vi "ToDatagram.vi"(8 "error in (no error)":errorcluster, 10 "messageID":u16, 11 "BaseMqttMsg in":refnum<class "BaseMqttMsg.lvclass">) -> (0 "error out":errorcluster, 2 "Datagram":u8[](array[numeric]), 3 "BaseMqttMsg out":refnum<class "BaseMqttMsg.lvclass">)   [LabVIEW 2020, in "BaseMqttMsg.lvclass"]
uses:
  BaseMqttMsg.lvclass
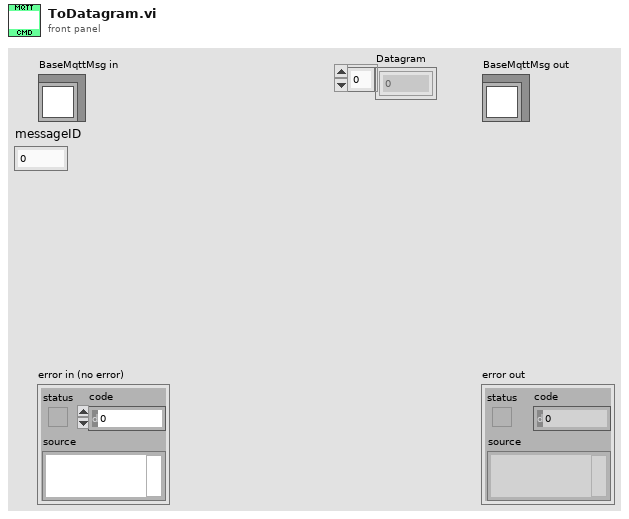
[diagram p1: front panel]
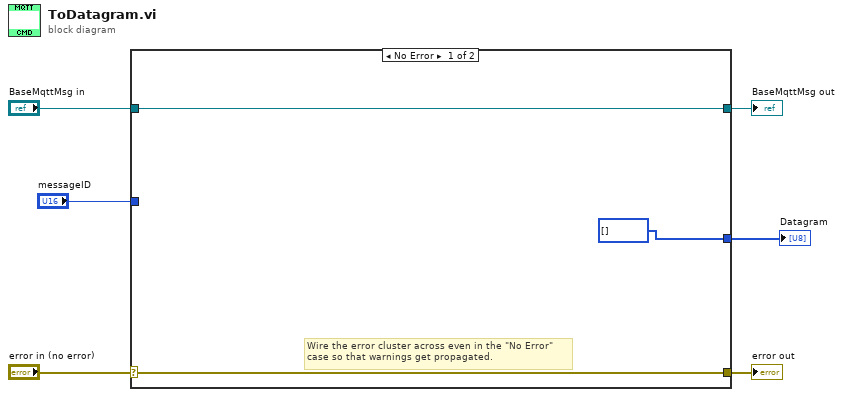
[diagram p0: block diagram]
diagram:
  n1 = case shown="No Error" "error in (no error)" {
    selector: "error in (no error)" -> [w8 w11]
    tunnel: [w8 w11] -> w5
    tunnel: [w9 w10] -> w3
    tunnel: "BaseMqttMsg in" -> [w9 w10]
    tunnel: [u8[] [] ("Datagram") _] -> w2
    tunnel: "messageID" -> [_ _]
    frame No Error {
      # "Wire the error cluster across even in the \"No Error\"\ncase so that warnings get propagated."
    }
    frame Error {
    }
  }
  "error out" <- w5
  "BaseMqttMsg out" <- w3
  "Datagram" <- w2
